vi "Vision Research Phantom Series PhCon PhNVMSaveClip.vi"(0 "CN in":u32=1, 1 "Cine":i32, 2 "pRng":T2, 3 "Options":T1 {"GI_HEADMASK" max=15}, 5 "Error In (no error)":errorcluster, 9 "CallID":u32) -> (14 "CN out":u32=1, 19 "Error Out":errorcluster)   [LabVIEW 2013, in "VRI.lvlib"]
doc: "PhCon.dll\n\nPhNVMSaveClip\nHRESULT PhNVMSaveClip(UINT CN, int Cine, PIMRANGE pRng, UINT Options, UINT CallID)\n\nParameters Description\nCN (in) Camera number.\nCine (in) Cine number.\npRng (in) Image range to be saved. NULL pointer means Save Full Cine.\nOptions (in) Uses GI_BPP16 to save the cine on 16 bits. If absent the bit depth will be 8 bits.\nCallID (in) The call identifier (a number 1 to 15). Used as a progress indicator parameter \n for calling PhLVProgress().\nReturn HRESULT (0 = Ok)\nComments Saves the cine recorded in DRAM to the NonVolatile memory (to the next free\n position). This saving does not depend on the range set by PhNVMSetRange."
uses:
  VRI.lvlib
  _Type Defs/PHCon IMRANGE.ctl
  _Type Defs/GetImage Options.ctl
  Phantom DLLs/PhCon.dll
panel:
  # "For instructions on the use of this VI, press Ctrl+H to display the help window and move the mouse over the icon, controls, and indicators"
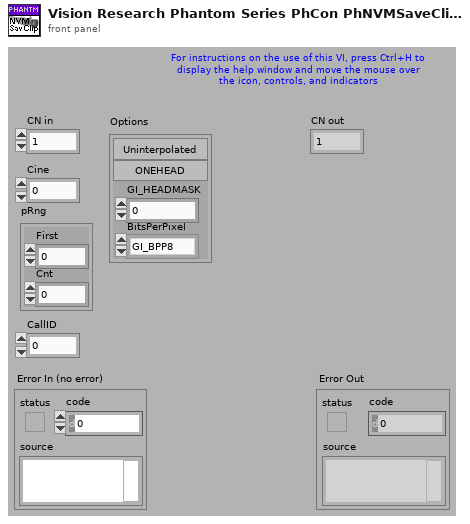
[diagram p1: front panel]
types:
  T1 = typedef "VRI.lvlib/GetImage Options.ctl" = cluster{"GI_INTERPOLATED":bool, "GI_ONEHEAD":bool, "GI_HEADMASK":u8, "BitsPerPixel":enum32{"GI_BPP8", "GI_PACKED", "GI_BPP16"}}
  T2 = typedef "VRI.lvlib/PHCon IMRANGE.ctl" = cluster{"First":i32, "Cnt":u32}
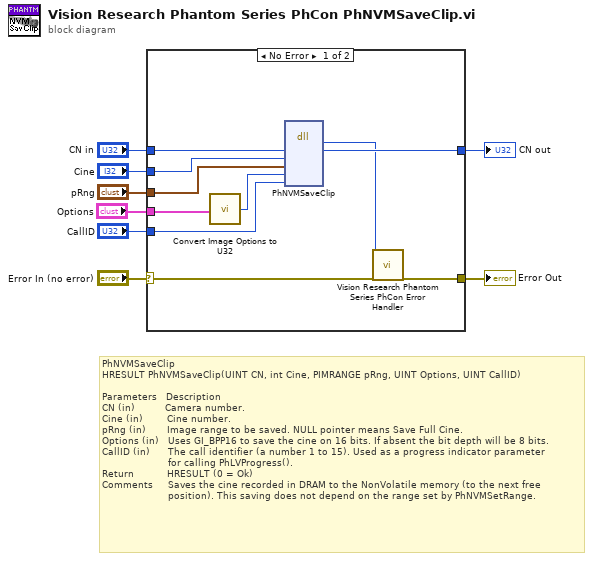
[diagram p0: block diagram]
diagram:
  # "PhNVMSaveClip\nHRESULT PhNVMSaveClip(UINT CN, int Cine, PIMRANGE pRng, UINT Options, UINT CallID)\n\nParameters   Description\nCN (in)          Camera number.\nCine (in)        Cine number.\npRng (in)       Image range to be saved. NULL pointer means Save Full Cine.\nOptions (in)   Uses GI_BPP16 to save the cine on 16 bits. If absent the bit depth will be 8 bits.\nCallID (in)      The call identifier (a number 1 to 15). Used as a progress indicator parameter \n                      for calling PhLVProgress().\nReturn           HRESULT (0 = Ok)\nComments     Saves the cine recorded in DRAM to the NonVolatile memory (to the next free\n                      position). This saving does not depend on the range set by PhNVMSetRange."
  n1 = case shown="No Error" "Error In (no error)" {
    selector: "Error In (no error)" -> [w18 w20]
    tunnel: [w17 w20] -> w7
    tunnel: "CN in" -> [w16 w19]
    tunnel: [w15 w19] -> w5
    tunnel: "Cine" -> [w14 _]
    tunnel: "pRng" -> [w13 _]
    tunnel: "Options" -> [w12 _]
    tunnel: "CallID" -> [w11 _]
    frame No Error {
      n2 = call "Convert Image Options to U32.vi"("Options"=w12) -> ("result"=w9:u32)
      n3 = dll-call lib="C:/Projects/SDK/32-bit/Vision Research Phantom Series Labview Driver/Phantom DLLs/PhCon.dll" fn="PhNVMSaveClip"("CN"=w16, "Cine"=w14, "pRng"=w13, "Options"=w9, "CallID"=w11) -> ("HRESULT"=w10:i32, "CN"=w15:u32)  [unwired: 7 in, 2 out]
      n4 = call "Vision Research Phantom Series PhCon Error Handler.vi"("ErrNo"=w10, "Error In (no error)"=w18) -> ("Error Out"=w17:errorcluster)  [unwired: 17 out]
    }
    frame Error {
    }
  }
  "Error Out" <- w7
  "CN out" <- w5
